vi "test averaging_filtering.vi"() -> ()   [LabVIEW 2014]
panel:
  out "averaging array":dbl[][](array[numeric])
  in  "?":i32=10000
  out "average and filter":cluster{cluster{dbl, "element":dbl}[]}[](graph)
  out "averaging":T1
  out "sum":dbl
  out "floor(x/y)":i32
  out "x-y*floor(x/y)":i32
  in  "average size":i32=5
  out "filtered + derivative":T1
  out "sum filtered":T1
  in  "raw":dbl[][](array[numeric])=array128x10000[1280000 elements]
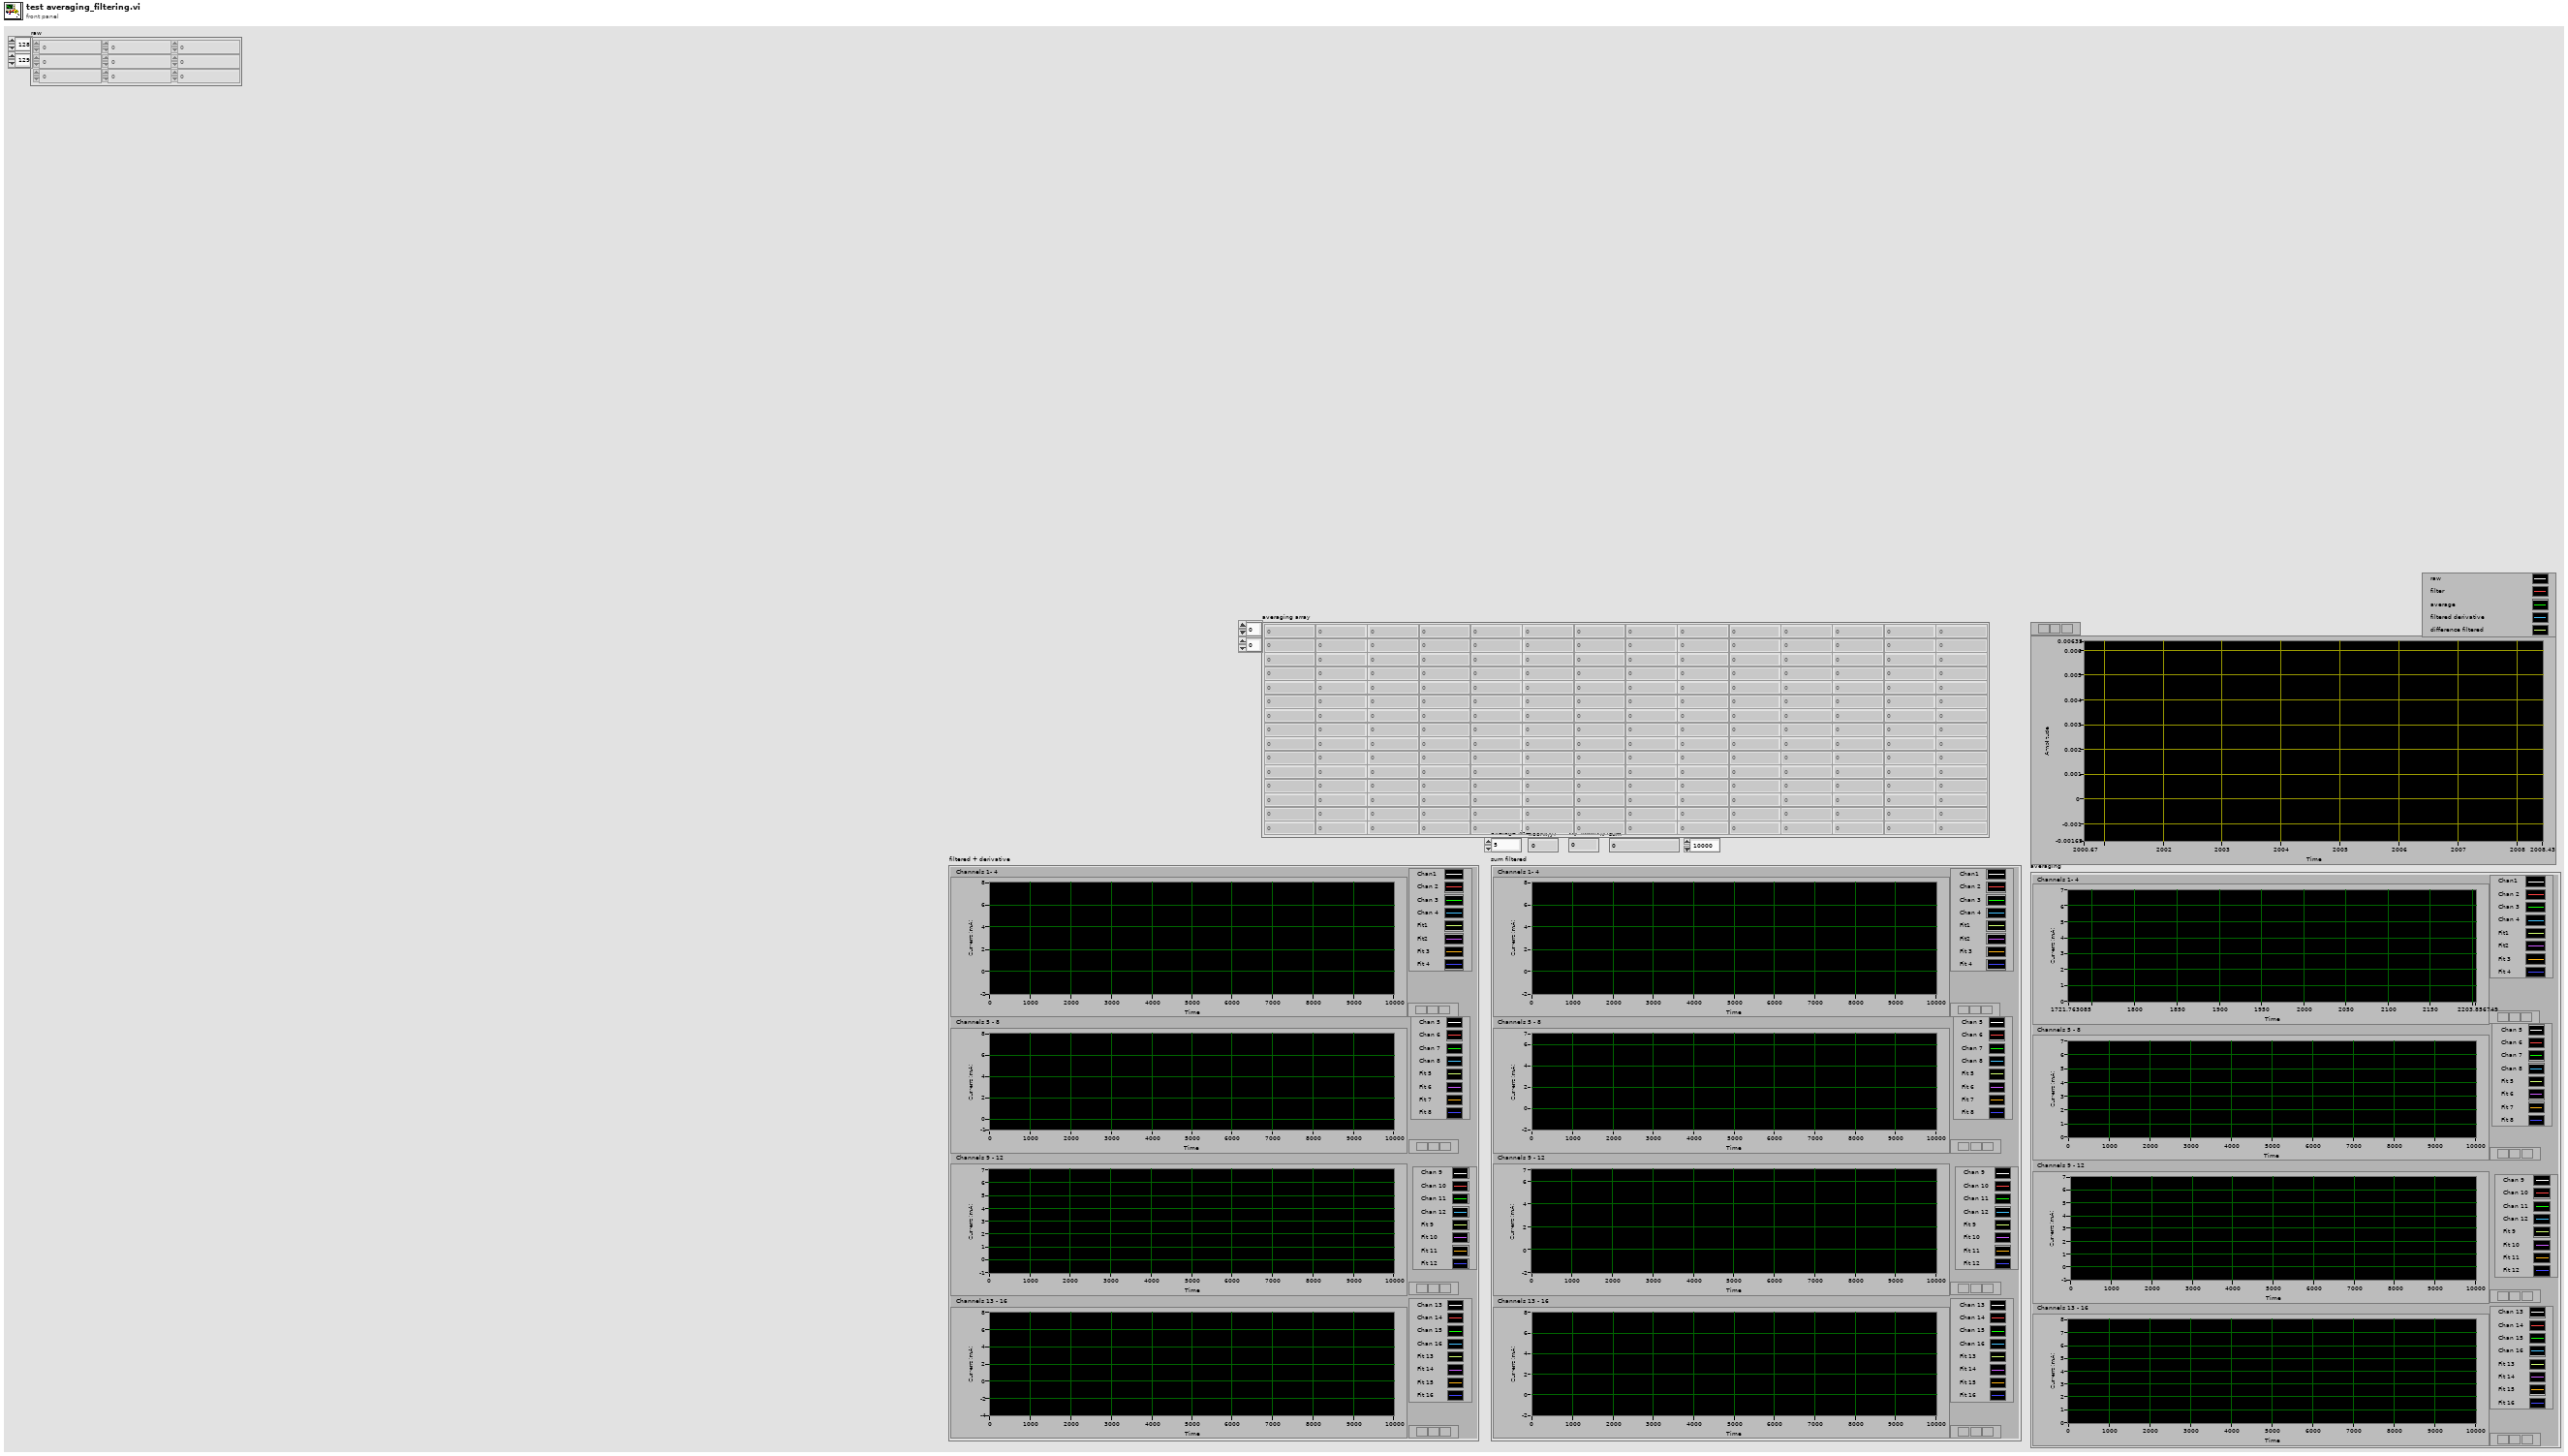
[diagram p1: front panel]
types:
  T1 = cluster{"Channels 1- 4":cluster{"tstart":sgl, "dt":sgl, "OutArray":dbl[][]}, "Channels 5 - 8":cluster{"tstart":sgl, "dt":sgl, "OutArray":dbl[][]}, "Channels 9 - 12":cluster{"tstart":sgl, "dt":sgl, "OutArray":dbl[][]}, "Channels 13 - 16":cluster{"tstart":sgl, "dt":sgl, "OutArray":dbl[][]}}
  T2 = cluster{"Channels 1- 8":cluster{"tstart":sgl, "dt":sgl, "OutArray":dbl[][]}, "Channels 9 - 16":cluster{"tstart":sgl, "dt":sgl, "OutArray":dbl[][]}, "Channels 17 - 24":cluster{"tstart":sgl, "dt":sgl, "OutArray":dbl[][]}, "Channels 25 - 32":cluster{"tstart":sgl, "dt":sgl, "OutArray":dbl[][]}}
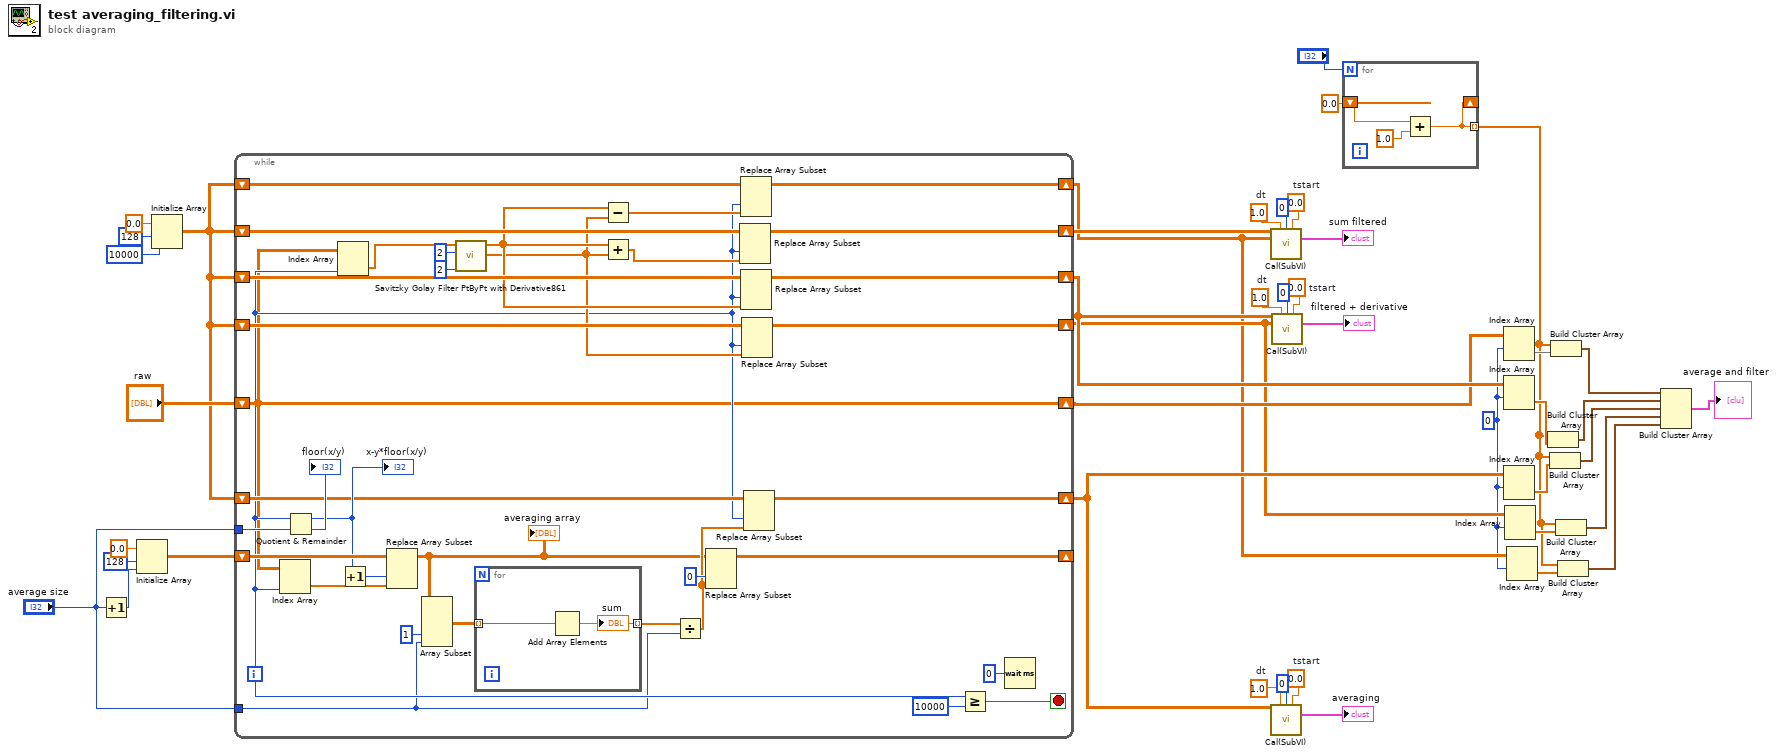
[diagram p0: block diagram]
diagram:
  w6 = 0 ("disabled index (col)")
  w23 = sgl 1.0  # dt
  w26 = sgl 0.0  # tstart
  w31 = sgl 1.0  # dt
  w33 = sgl 0.0  # tstart
  w39 = sgl 1.0  # dt
  w41 = sgl 0.0  # tstart
  n1 = Increment(x="average size") -> (x+1=w10:i32)
  n2 = Initialize Array(0.0 ("element"), 128 ("dimension size"), w10) -> (w28:dbl[][])
  n3 = Initialize Array(0.0 ("element"), 128 ("dimension size"), 10000 ("dimension size")) -> (w24:dbl[][])
  n4 = while {
    shift-right: [w72] -> w35
    shift-left: w24 -> [w73]
    shift-right: [w67] -> w8
    shift-left: w24 -> [w69]
    shift-right: [w68] -> w17
    shift-left: w24 -> [w70]
    shift-right: [w62] -> w7
    shift-left: w24 -> [w64]
    shift-right: [w54] -> _
    shift-left: w28 -> [w59]
    tunnel: "average size" -> [w61]
    shift-right: [w51] -> w16
    shift-left: w24 -> [w53]
    tunnel: "average size" -> [w45]
    shift-right: [w44] -> w13
    shift-left: "raw" -> [w44]
    i -> [w52]
    stop <- w76 stop-if-true
    n5 = Index Array(array=w44, index (col)=w52) -> (element=w58:dbl[])  [unwired: 1 in]
    n6 = Quotient & Remainder(x=w52, y=w61) -> (x-y*floor(x/y)=w57:i32, floor(x/y)=→"floor(x/y)":i32)
    "x-y*floor(x/y)" <- w57
    n7 = Index Array(array=w44, index (col)=w52) -> (element=w75:dbl[])  [unwired: 1 in]
    n8 = Increment(x=w57) -> (x+1=w56:i32)
    n9 = Replace Array Subset(array=w59, new element=w58, index (col)=w56) -> (w47:dbl[][])  [unwired: 1 in]
    "averaging array" <- w47
    n10 = Array Subset(array=w47, index (col)=1 ("index"), length (col)=w45) -> (w48:dbl[][])  [unwired: 2 in]
    n11 = call "Savitzky Golay Filter PtByPt with Derivative861.vi"("order polynomial"=2, "side points"=2, "x"=w75) -> ("Filtered Derivative"=w65:dbl[], "Filtered x"=w66:dbl[])  [unwired: 1 in, 6 out]
    n12 = for {
      tunnel: w48 -> [w81] mode=indexing
      tunnel: [w80] -> w50 mode=indexing
      n13 = Add Array Elements(numeric array=w81) -> (sum=w80:dbl)
      "sum" <- w80
    }
    n14 = Subtract(x=w66, y=w65) -> (x-y=w63:dbl[])
    n15 = Add(x=w66, y=w65) -> (x+y=w71:dbl[])
    n16 = Divide(x=w50, y=w45) -> (x/y=w49:dbl[])
    n17 = Replace Array Subset(array=w47, new element=w49, index (col)=0 ("disabled index (col)")) -> (w54:dbl[][])  [unwired: 1 in]
    n18 = Replace Array Subset(array=w73, new element=w71, index (col)=w52) -> (w72:dbl[][])  [unwired: 1 in]
    n19 = Replace Array Subset(array=w64, new element=w63, index (col)=w52) -> (w62:dbl[][])  [unwired: 1 in]
    n20 = Replace Array Subset(array=w70, new element=w66, index (col)=w52) -> (w68:dbl[][])  [unwired: 1 in]
    n21 = Replace Array Subset(array=w69, new element=w65, index (col)=w52) -> (w67:dbl[][])  [unwired: 1 in]
    n22 = Replace Array Subset(array=w53, new element=w49, index (col)=w52) -> (w51:dbl[][])  [unwired: 1 in]
    n23 = Greater Or Equal?(x=w52, y=10000) -> (x >= y?=w76:bool)
    n24 = Wait (ms)(milliseconds to wait=u32 0) -> ()  [unwired: 1 out]
  }
  n25 = call "Cal(SubVI).vi"("Array"=w35, "dt"=w39, "StartChan"=0 ("ChanStart"), "tstart"=w41, "FitData"=w7) -> ("plot(Signals) 1-32"=→"sum filtered":T2)  [unwired: 9 in, 1 out]
  n26 = call "Cal(SubVI).vi"("Array"=w16, "dt"=w23, "StartChan"=0 ("ChanStart"), "tstart"=w26) -> ("plot(Signals) 1-32"=→"averaging":T2)  [unwired: 10 in, 1 out]
  n27 = call "Cal(SubVI).vi"("Array"=w17, "dt"=w31, "StartChan"=0 ("ChanStart"), "tstart"=w33, "FitData"=w8) -> ("plot(Signals) 1-32"=→"filtered + derivative":T2)  [unwired: 9 in, 1 out]
  n28 = for {
    N: "?" -> [_]
    tunnel: [w84] -> w3 mode=indexing
    shift-right: [w84] -> _
    shift-left: 0.0 -> [w83]
    n29 = Add(x=w83, y=1.0 ("TimeStep")) -> (x+y=w84:dbl)
  }
  n30 = Index Array(array=w13, index (row)=w6) -> (element=w12:dbl[])  [unwired: 1 in]
  n31 = Index Array(array=w17, index (row)=w6) -> (element=w20:dbl[])  [unwired: 1 in]
  n32 = Index Array(array=w16, index (row)=w6) -> (element=w19:dbl[])  [unwired: 1 in]
  n33 = Index Array(array=w8, index (row)=w6) -> (element=w5:dbl[])  [unwired: 1 in]
  n34 = Index Array(array=w7, index (row)=w6) -> (element=w4:dbl[])  [unwired: 1 in]
  n35 = Build Cluster Array(w3, w20) -> (w21:cluster{dbl, "element":dbl}[])
  n36 = Build Cluster Array(w3, w19) -> (w18:cluster{dbl, "element":dbl}[])
  n37 = Build Cluster Array(w3, w12) -> (w11:cluster{dbl, dbl}[])
  n38 = Build Cluster Array(w3, w5) -> (w2:cluster{dbl, "element":dbl}[])
  n39 = Build Cluster Array(w3, w4) -> (w1:cluster{dbl, "element":dbl}[])
  n40 = Build Cluster Array(w11, w21, w18, w2, w1) -> (→"average and filter":cluster{cluster{dbl, "element":dbl}[]}[])
